vi "Clear DAQ Multi IO.vi"(8 "error in":errorcluster, 11 "DAQ Ref":T1) -> (0 "error out":errorcluster)   [LabVIEW 2021]
uses:
  Controls/DAQ Refnums.ctl
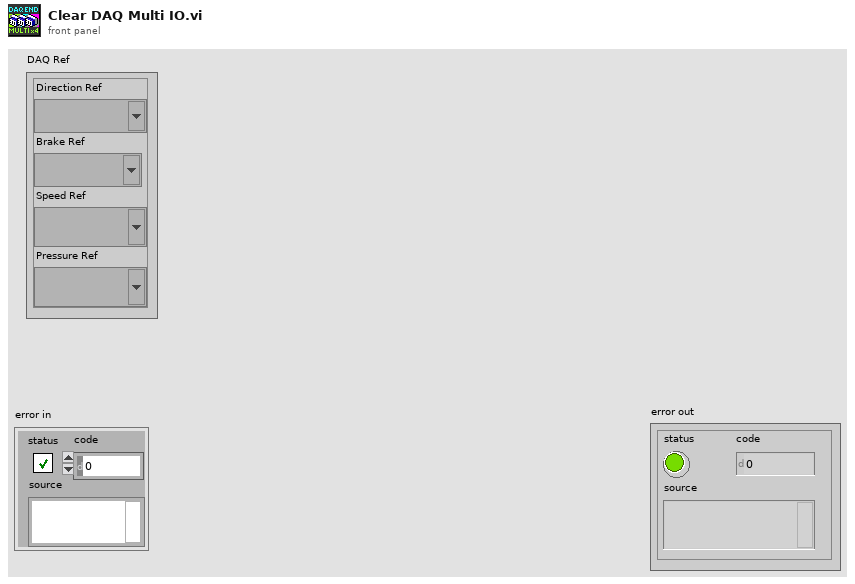
[diagram p1: front panel]
types:
  T1 = typedef "DAQ Refnums.ctl" = cluster{"Direction Ref":refnum<k21>, "Brake Ref":refnum<k21>, "Speed Ref":refnum<k21>, "Pressure Ref":refnum<k21>}
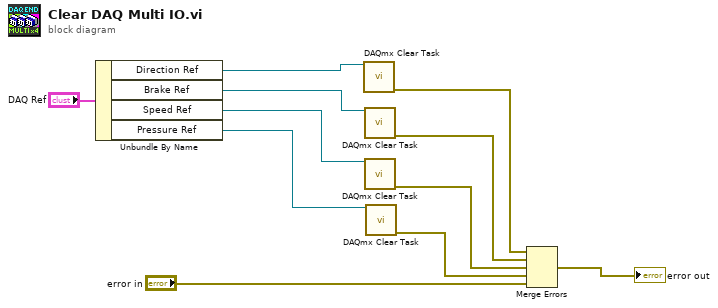
[diagram p0: block diagram]
diagram:
  n1 = Unbundle By Name("DAQ Ref") -> ("Direction Ref"=w2:refnum<k21>, "Brake Ref"=w5:refnum<k21>, "Speed Ref"=w4:refnum<k21>, "Pressure Ref"=w3:refnum<k21>)
  n2 = call <vilib>:"DAQmx Clear Task.vi"("task in"=w2) -> ("error out"=w6:errorcluster)  [unwired: 14 in]
  n3 = call <vilib>:"DAQmx Clear Task.vi"("task in"=w5) -> ("error out"=w7:errorcluster)  [unwired: 14 in]
  n4 = call <vilib>:"DAQmx Clear Task.vi"("task in"=w4) -> ("error out"=w8:errorcluster)  [unwired: 14 in]
  n5 = call <vilib>:"DAQmx Clear Task.vi"("task in"=w3) -> ("error out"=w9:errorcluster)  [unwired: 14 in]
  n6 = Merge Errors(w6, w7, w8, w9, "error in") -> (→"error out":errorcluster)
